vi "Array Subset by Value.vi"(9 "End":dbl=2000000.0 format="%#_6p", 10 "Start":dbl=500000.0 format="%#_6p", 11 "Data":dbl[](array[numeric])) -> (3 "Data subset":dbl[](array[numeric]))   [LabVIEW 2019]
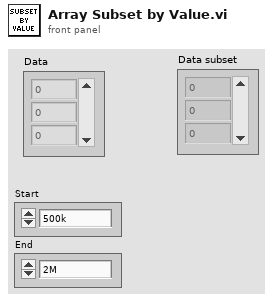
[diagram p1: front panel]
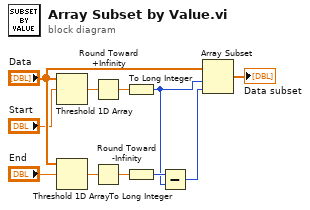
[diagram p0: block diagram]
diagram:
  n1 = Threshold 1D Array(2:"Start", 3:"Data") -> (0:w11:dbl)  [unwired: 1 in]
  n2 = Threshold 1D Array(2:"End", 3:"Data") -> (0:w10:dbl)  [unwired: 1 in]
  n3 = Round Toward +Infinity(x=w11) -> (ceil(x): smallest int >= x=w9:dbl)
  n4 = Round Toward -Infinity(1:w10) -> (0:w8:dbl)
  n5 = To Long Integer(number=w9) -> (32bit integer=w6:i32)
  n6 = To Long Integer(number=w8) -> (32bit integer=w7:i32)
  n7 = Subtract(x=w7, y=w6) -> (x-y=w5:i32)
  n8 = Array Subset(array="Data", index=w6, length=w5) -> (→"Data subset":dbl[])
